vi "PMU_DATA_PACK.vi"(0 "DATA FRAME":string, 2 "DATA_IN":T2, 3 "PMUs_NUM":u16) -> (6 "PMU DATA Packet":string[](array[string]), 9 "DATA_DTLD":T1, 10 "STAT FIELD":string[](array[string]))   [LabVIEW 2013]
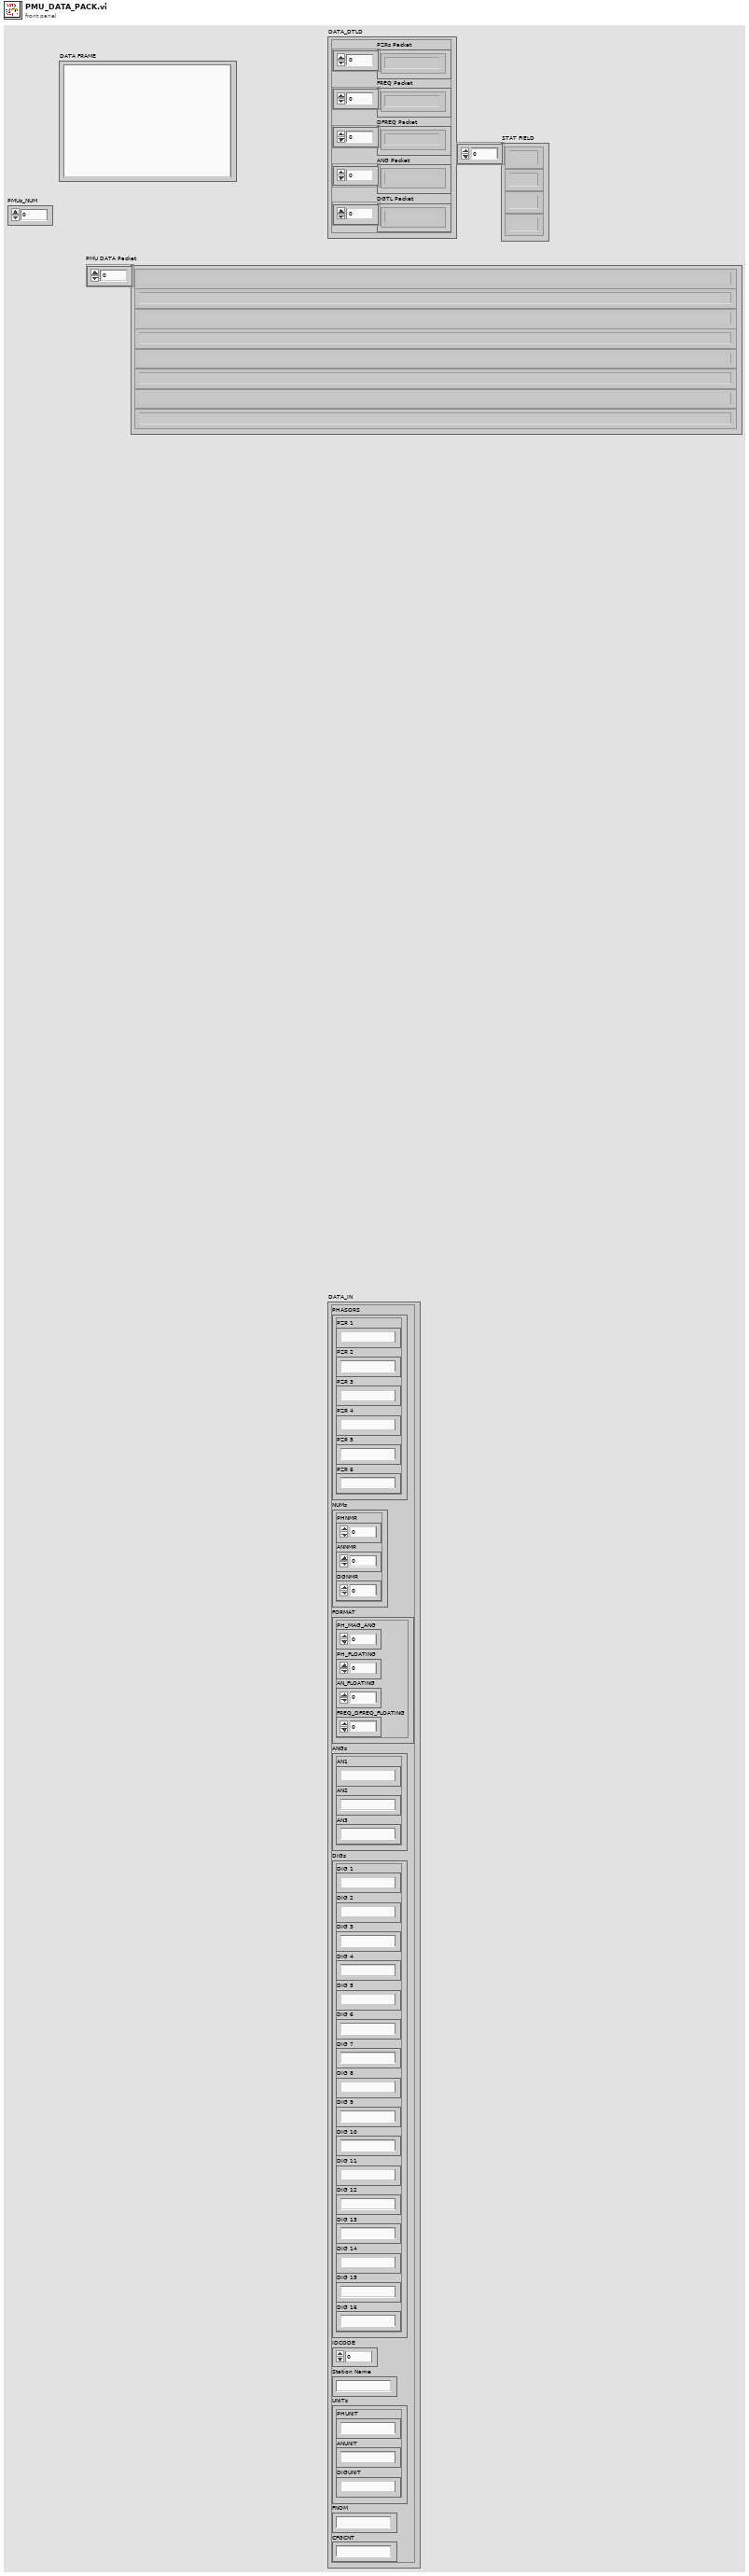
[diagram p1: front panel]
types:
  T1 = cluster{"PZRs Packet":string[], "FREQ Packet":string[], "DFREQ Packet":string[], "ANG Packet":string[], "DGTL Packet":string[]}
  T2 = cluster{"PHASORS":cluster{"PZR 1":string, "PZR 2":string, "PZR 3":string, "PZR 4":string, "PZR 5":string, "PZR 6":string}, "NUMs":cluster{"PHNMR":u8, "ANNMR":u8, "DGNMR":u8}, "FORMAT":cluster{"PH_MAG_ANG":u16, "PH_FLOATING":u16, "AN_FLOATING":u16, "FREQ_DFREQ_FLOATING":u16}, "ANGs":cluster{"AN1":string, "AN2":string, "AN3":string}, "DIGs":cluster{"DIG 1":string, "DIG 2":string, "DIG 3":string, "DIG 4":string, "DIG 5":string, "DIG 6":string, "DIG 7":string, "DIG 8":string, "DIG 9":string, "DIG 10":string, "DIG 11":string, "DIG 12":string, "DIG 13":string, "DIG 14":string, "DIG 15":string, "DIG 16":string}, "IDCODE":u16, "Station Name":string, "UNITs":cluster{"PHUNIT":string, "ANUNIT":string, "DIGUNIT":string}, "FNOM":string, "CFGCNT":string}
  T3 = cluster{"PH_MAG_ANG":u16, "PH_FLOATING":u16, "AN_FLOATING":u16, "FREQ_DFREQ_FLOATING":u16}
  T4 = cluster{"PHNUMR":u16, "ANNUMR":u16, "DGNUMR":u16}
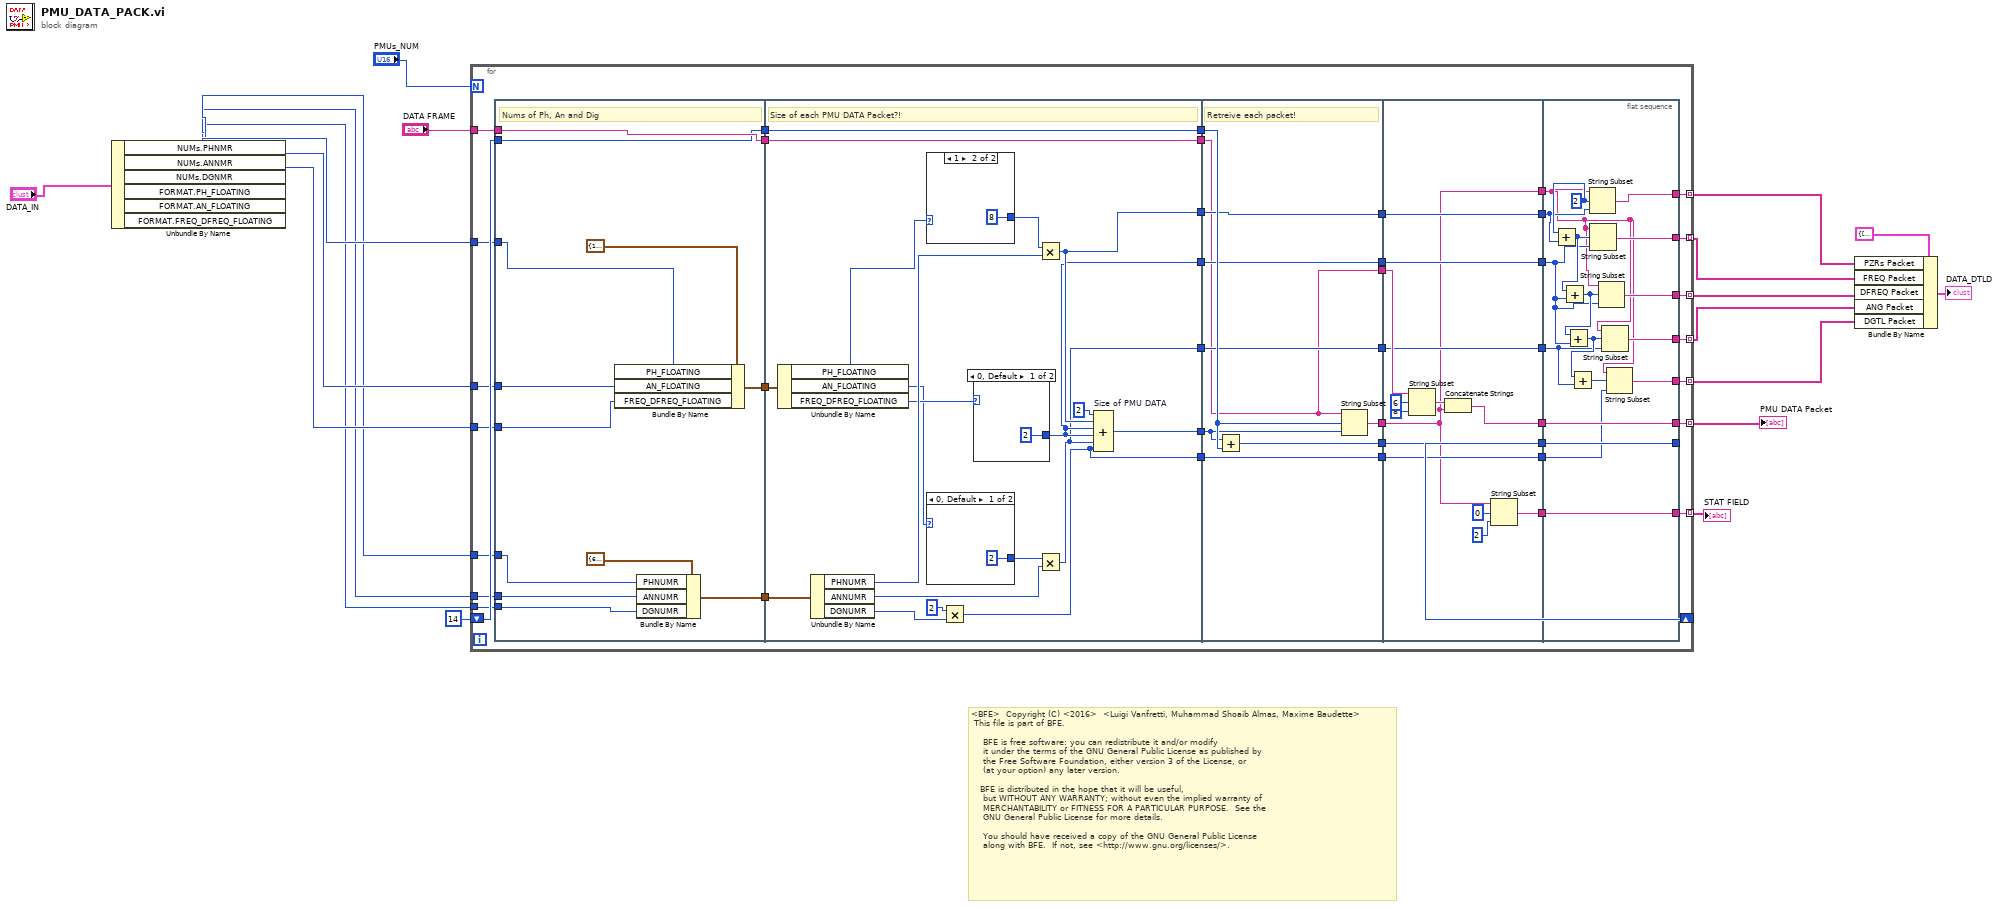
[diagram p0: block diagram]
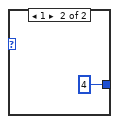
[diagram p2: hidden frame]
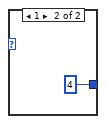
[diagram p3: hidden frame]
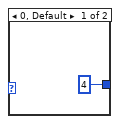
[diagram p4: hidden frame]
diagram:
  # "<BFE>  Copyright (C) <2016>  <Luigi Vanfretti, Muhammad Shoaib Almas, Maxime Baudette>\n This file is part of BFE.\n\n    BFE is free software: you can redistribute it and/or modify\n    it under the terms of the GNU General Public License as published by\n    the Free Software Foundation, either version 3 of the License, or\n    (at your option) any later version.\n\n   BFE is distributed in the hope that it will be useful,\n    but WITHOUT ANY WARRANTY; without even the implied warranty of\n    MERCHANTABILITY or FITNESS FOR A PARTICULAR PURPOSE.  See the\n    GNU General Public License for more details.\n\n    You should have received a copy of the GNU General Public License\n    along with BFE.  If not, see <http://www.gnu.org/licenses/>."
  n1 = Unbundle By Name("DATA_IN") -> ("NUMs.PHNMR"=w12:u8, "NUMs.ANNMR"=w11:u8, "NUMs.DGNMR"=w10:u8, "FORMAT.PH_FLOATING"=w15:u16, "FORMAT.AN_FLOATING"=w14:u16, "FORMAT.FREQ_DFREQ_FLOATING"=w13:u16)
  n2 = for {
    N: "PMUs_NUM" -> [_]
    tunnel: "DATA FRAME" -> [w61]
    shift-right: [w53] -> _
    shift-left: 14 -> [w54]
    tunnel: [w52] -> w18 mode=indexing
    tunnel: w12 -> [w51]
    tunnel: w11 -> [w50]
    tunnel: w10 -> [w49]
    tunnel: w15 -> [w48]
    tunnel: w14 -> [w46]
    tunnel: w13 -> [w45]
    tunnel: [w38] -> w8 mode=indexing
    tunnel: [w34] -> w7 mode=indexing
    tunnel: [w30] -> w6 mode=indexing
    tunnel: [w26] -> w5 mode=indexing
    tunnel: [w25] -> w4 mode=indexing
    tunnel: [w21] -> w1 mode=indexing
    n3 = flat-sequence {
      tunnel: w61 -> [w71]
      tunnel: [w72] -> w60
      tunnel: [w71] -> w58
      tunnel: [w70] -> w55
      tunnel: w54 -> [w70]
      tunnel: w51 -> [w69]
      tunnel: w50 -> [w68]
      tunnel: w49 -> [w67]
      tunnel: w48 -> [w64]
      tunnel: [w65] -> w47
      tunnel: w46 -> [w63]
      tunnel: w45 -> [w62]
      tunnel: w60 -> [w92]
      tunnel: [w91] -> w59
      tunnel: w58 -> [w91]
      tunnel: [w89] -> w57
      tunnel: [w90] -> w56
      tunnel: w55 -> [w90]
      tunnel: w47 -> [w85]
      tunnel: [w77] -> w35
      tunnel: [w76] -> w33
      tunnel: [w75] -> w29
      tunnel: [w74] -> w24
      tunnel: w59 -> [w99]
      tunnel: w57 -> [w104]
      tunnel: w56 -> [w106]
      tunnel: [w105] -> w44
      tunnel: [w107] -> w43
      tunnel: [w99] -> w42
      tunnel: [w103] -> w36
      tunnel: w35 -> [w103]
      tunnel: w33 -> [w102]
      tunnel: [w102] -> w32
      tunnel: w29 -> [w101]
      tunnel: [w101] -> w28
      tunnel: w24 -> [w100]
      tunnel: [w100] -> w23
      tunnel: w44 -> [w121]
      tunnel: w43 -> [w109]
      tunnel: w42 -> [w120]
      tunnel: [w121] -> w41
      tunnel: [w118] -> w40
      tunnel: [w109] -> w39
      tunnel: [w115] -> w37
      tunnel: w36 -> [w115]
      tunnel: w32 -> [w114]
      tunnel: [w114] -> w31
      tunnel: w28 -> [w113]
      tunnel: [w113] -> w27
      tunnel: w23 -> [w112]
      tunnel: [w112] -> w22
      tunnel: [w108] -> w20
      tunnel: [w138] -> w52
      tunnel: [w139] -> w53
      tunnel: w41 -> [w139]
      tunnel: w40 -> [w138]
      tunnel: w39 -> [w123]
      tunnel: [w137] -> w38
      tunnel: w37 -> [w134]
      tunnel: [w136] -> w34
      tunnel: w31 -> [w130]
      tunnel: [w132] -> w30
      tunnel: w27 -> [w126]
      tunnel: [w129] -> w26
      tunnel: [w125] -> w25
      tunnel: w22 -> [w124]
      tunnel: [w122] -> w21
      tunnel: w20 -> [w122]
      frame #0 {
        # "Nums of Ph, An and Dig"
        n4 = Bundle By Name(cluster=T3 {"PH_MAG_ANG"=1, "PH_FLOATING"=2, "AN_FLOATING"=4, "FREQ_DFREQ_FLOATING"=8}, "PH_FLOATING"=w64, "AN_FLOATING"=w63, "FREQ_DFREQ_FLOATING"=w62) -> (w65:T3)
        n5 = Bundle By Name(cluster=T4 {"PHNUMR"=6, "ANNUMR"=3, "DGNUMR"=1}, "PHNUMR"=w69, "ANNUMR"=w68, "DGNUMR"=w67) -> (w72:T4)
      }
      frame #1 {
        # "Size of each PMU DATA Packet?!"
        n6 = Unbundle By Name(w85) -> ("PH_FLOATING"=w84:u16, "AN_FLOATING"=w82:u16, "FREQ_DFREQ_FLOATING"=w83:u16)
        n7 = Unbundle By Name(w92) -> ("PHNUMR"=w86:u16, "ANNUMR"=w80:u16, "DGNUMR"=w78:u16)
        n8 = case shown="1" w84 {
          tunnel: [u8 4 ("value") u8 8 ("value")] -> w87
          frame 0, Default {
          }
          frame 1 {
          }
        }
        n9 = case shown="0, Default" w82 {
          tunnel: [u8 2 ("value") u8 4 ("value")] -> w81
          frame 0, Default {
          }
          frame 1 {
          }
        }
        n10 = Multiply(x=u8 2 ("value"), y=w78) -> (x*y=w74:u16)
        n11 = case shown="0, Default" w83 {
          tunnel: [u8 2 ("value") u8 4 ("value")] -> w76
          frame 0, Default {
          }
          frame 1 {
          }
        }
        n12 = Multiply(x=w87, y=w86) -> (x*y=w77:u16)
        n13 = Multiply(x=w81, y=w80) -> (x*y=w75:u16)
        n14 = Compound Arithmetic op=ADD "Size of PMU DATA"(u8 2 ("value"), w77, w76, w76, w75, w74) -> (w89:u16)
      }
      frame #2 {
        # "Retreive each packet!"
        n15 = Add(x=w104, y=w106) -> (x+y=w105:i32)
        n16 = String Subset(string=w99, offset (0)=w106, length (rest)=w104) -> (substring=w107:string)
      }
      frame #3 {
        n17 = String Subset(string=w120, offset (0)=6, length (rest)=8 ("length (rest)")) -> (substring=w119:string)
        n18 = Concatenate Strings(w119, w109) -> (w118:string)
        n19 = String Subset(string=w109, offset (0)=0, length (rest)=2 ("length (rest)")) -> (substring=w108:string)
      }
      frame #4 {
        w135 = 2 ("offset (0)")
        n20 = Add(x=w135, y=w134) -> (x+y=w133:i32)
        n21 = Add(x=w133, y=w130) -> (x+y=w131:i32)
        n22 = Add(x=w131, y=w130) -> (x+y=w127:i32)
        n23 = Add(x=w127, y=w126) -> (x+y=w128:i32)
        n24 = String Subset(string=w123, offset (0)=w135, length (rest)=w134) -> (substring=w137:string)
        n25 = String Subset(string=w123, offset (0)=w133, length (rest)=w130) -> (substring=w136:string)
        n26 = String Subset(string=w123, offset (0)=w131, length (rest)=w130) -> (substring=w132:string)
        n27 = String Subset(string=w123, offset (0)=w127, length (rest)=w126) -> (substring=w129:string)
        n28 = String Subset(string=w123, offset (0)=w128, length (rest)=w124) -> (substring=w125:string)
      }
    }
  }
  "PMU DATA Packet" <- w18
  "STAT FIELD" <- w1
  n29 = Bundle By Name(cluster=T1 {"PZRs Packet"=[], "FREQ Packet"=[], "DFREQ Packet"=[], "ANG Packet"=[], "DGTL Packet"=[]}, "PZRs Packet"=w8, "FREQ Packet"=w7, "DFREQ Packet"=w6, "ANG Packet"=w5, "DGTL Packet"=w4) -> (→"DATA_DTLD":T1)
